vi "InitPluginIndex.vi"(8 "ErrorArray":errorcluster[](array[cluster]), 10 "RingRefArray":refnum<vi>[](array[refnum]), 11 "TestBase in":refnum<class "TestBase.lvclass">) -> (0 "ErrorArray":errorcluster[](array[cluster]), 3 "TestBase out":refnum<class "TestBase.lvclass">)   [LabVIEW 2014, in "TestBase.lvclass"]
uses:
  TestBase.lvclass
  TestBase.lvclass/TestBase.ctl
  Accessors/Write PluginIndex.vi
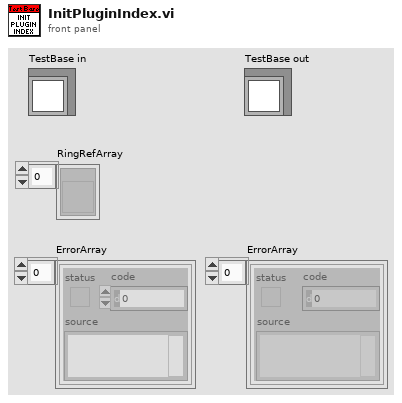
[diagram p1: front panel]
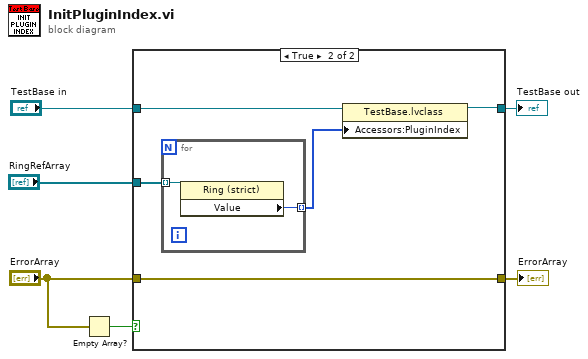
[diagram p0: block diagram]
diagram:
  n1 = Empty Array?(array="ErrorArray") -> (empty?=w3:bool)
  n2 = case shown="True" w3 {
    tunnel: [w8 w9] -> w5
    tunnel: "TestBase in" -> [w8 w13]
    tunnel: "RingRefArray" -> [_ w12]
    tunnel: [w7 w10] -> w1
    tunnel: "ErrorArray" -> [w7 w10]
    frame False {
    }
    frame True {
      n3 = for {
        tunnel: w12 -> [w15] mode=indexing
        tunnel: [w14] -> w11 mode=indexing
        n4 = property class="Ring (strict)"(reference=w15) -> ("Value"=w14:u16)  [unwired: 1 in, 2 out]
      }
      n5 = property class="TestBase.lvclass"(reference=w13, "Accessors:PluginIndex"=w11) -> (reference out=w9:refnum<class "TestBase.lvclass">)  [unwired: 1 in, 1 out]
    }
  }
  "TestBase out" <- w5
  "ErrorArray" <- w1
